vi "append string test.vi"() -> ()   [LabVIEW 2019]
uses:
  <vilib>/JKI/JKI SMO/SMO/Typedefs/SMOState --Enum.ctl
  <userlib>/_OpenG.lib/string/string.llb/Trim Whitespace (String)__ogtk.vi
  <vilib>/JKI/JKI SMO/SMO/SMO.lvclass
panel:
  out "resulting string":string
  in  "SMO State 2":T1
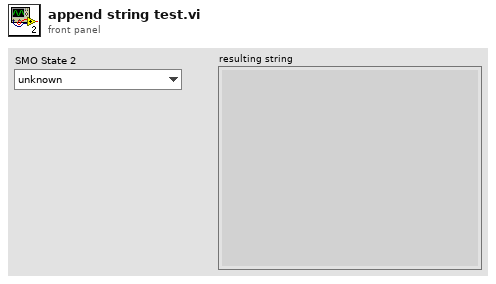
[diagram p1: front panel]
types:
  T1 = typedef "SMO.lvclass/SMOState --Enum.ctl" = enum16{"unknown", "Created", "Started", "Stopped"}
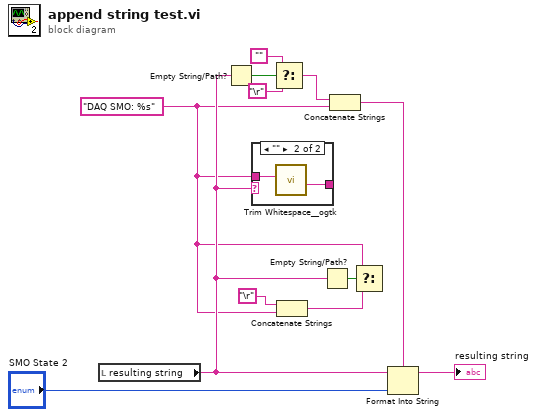
[diagram p0: block diagram]
diagram:
  w5 = "DAQ SMO: %s" ("format string")
  n1 = local read "resulting string"() -> (w7:string)
  n2 = Empty String/Path?(string/path=w7) -> (empty?=w6:bool)
  n3 = case shown="\"\"" w7 {
    tunnel: w5 -> [w13 w15]
    tunnel: [w13 w14] -> _
    frame Default {
    }
    frame "" {
      n4 = call-poly <userlib>:"Trim Whitespace__ogtk.vi"("String in"=w15) -> ("String out"=w14:string)  [unwired: 6 in]
    }
  }
  n5 = Select(t="", s=w6, f="\r") -> (s? t:f=w3:string)
  n6 = Concatenate Strings("\r", w5) -> (w9:string)
  n7 = Empty String/Path?(string/path=w7) -> (empty?=w10:bool)
  n8 = Concatenate Strings(w3, w5) -> (w4:string)
  n9 = Select(t=w5, s=w10, f=w9) -> ()  [unwired: 1 out]
  n10 = Format Into String(format string=w4, initial string=w7, "SMO State 2") -> (resulting string=→"resulting string":string)  [unwired: 1 in, 1 out]
